vi "Library Data FGV.vi"(8 "error in (no error)":errorcluster, 10 "FGV Actions":T1, 11 "Library Information in":T2={"Right Motor Name"="", "Left Motor Name"="", "Current Control Mode"=7, "Motion Magic Parameters"={"Native Units"=0.0}, "Motor Controllers Parameters"={"Max Current (amps)"=0, "PID Buckets"={"High Gear"=0, "High Gear Ramp"=0, "Low Gear"=0, "Low Gear Ramp"=0}}} {"Current Control Mode" items=["PercentOutput"=0, "Position"=1, "Velocity"=2, "Current"=3, "Follower"=5, "MotionProfile"=6, "MotionMagic"=7, "MotionMagicArc"=8, "MotionProfileArc"=10, "Disabled"=15]}) -> (0 "error out":errorcluster, 3 "Library Information out":T2={"Right Motor Name"="", "Left Motor Name"="", "Current Control Mode"=7, "Motion Magic Parameters"={"Native Units"=0.0}, "Motor Controllers Parameters"={"Max Current (amps)"=0, "PID Buckets"={"High Gear"=0, "High Gear Ramp"=0, "Low Gear"=0, "Low Gear Ramp"=0}}} {"Current Control Mode" items=["PercentOutput"=0, "Position"=1, "Velocity"=2, "Current"=3, "Follower"=5, "MotionProfile"=6, "MotionMagic"=7, "MotionMagicArc"=8, "MotionProfileArc"=10, "Disabled"=15]})   [LabVIEW 2017, in "Drive Train.lvlib"]
uses:
  Drive Train.lvlib
  Controls/Library Information.ctl
  <vilib>/Rock Robotics/WPI/ThirdParty/Phoenix-LabVIEW/Motor Controller/Controls/CTRE_Phoenix_MotorControl_ControlMode.ctl
  Controls/Motion Magic Parameters.ctl
  Controls/Motor Controllers Parameters.ctl
  Controls/FGV Actions.ctl
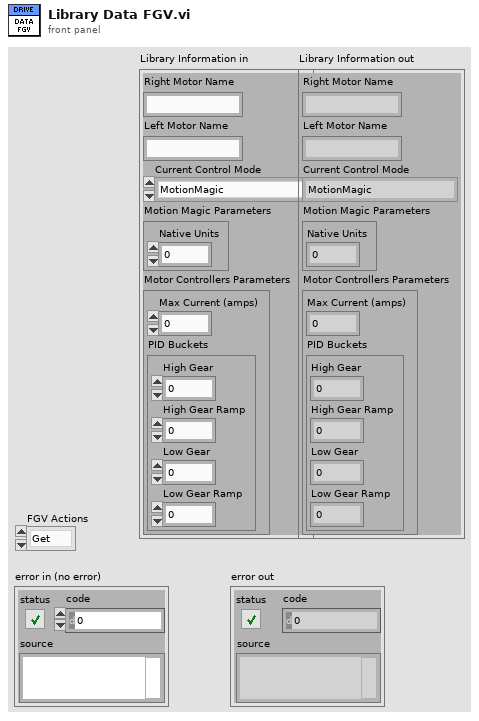
[diagram p1: front panel]
types:
  T1 = typedef "Drive Train.lvlib/FGV Actions.ctl" = enum16{"Get", "Set"}
  T2 = typedef "Drive Train.lvlib/Library Information.ctl" = cluster{"Right Motor Name":string, "Left Motor Name":string, "Current Control Mode":T3, "Motion Magic Parameters":T4, "Motor Controllers Parameters":T5}
  T3 = typedef "CTRE_Phoenix_MotorControl_ControlMode.ctl" = u16
  T4 = typedef "Drive Train.lvlib/Motion Magic Parameters.ctl" = cluster{"Native Units":dbl}
  T5 = typedef "Drive Train.lvlib/Motor Controllers Parameters.ctl" = cluster{"Max Current (amps)":i32, "PID Buckets":cluster{"High Gear":i32, "High Gear Ramp":i32, "Low Gear":i32, "Low Gear Ramp":i32}}
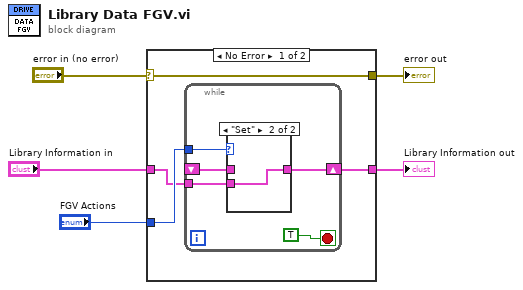
[diagram p0: block diagram]
diagram:
  n1 = case shown="No Error" "error in (no error)" {
    selector: "error in (no error)" -> [w9 w18]
    tunnel: [w9 w18] -> w4
    tunnel: "Library Information in" -> [w6 w17]
    tunnel: [w8 w17] -> w2
    tunnel: "FGV Actions" -> [w7 _]
    frame No Error {
      n2 = while {
        shift-right: [w12] -> w8
        shift-left: _ -> [w11]
        tunnel: w7 -> [w13]
        tunnel: w6 -> [w10]
        stop <- TRUE stop-if-true
        n3 = case shown="\"Set\"" w13 {
          tunnel: [w15 w16] -> w12
          tunnel: w11 -> [w15 _]
          tunnel: w10 -> [_ w16]
          frame "Get", Default {
          }
          frame "Set" {
          }
        }
      }
    }
    frame Error {
    }
  }
  "Library Information out" <- w2
  "error out" <- w4
